vi "多路CAN初始化.vi"(8 "错误输入（无错误）":errorcluster, 11 "CAN通道in":u16[](array[numeric])=[81, 82, 83]) -> (0 "错误out（无错误）":errorcluster caption="错误输入（无错误）", 3 "CAN 通道out":u16[](array[numeric]))   [LabVIEW 2020]
uses:
  <userlib>/PCANBasic/PCANBasic.lvlib
panel:
  out "function return":u32 format="%.0x"
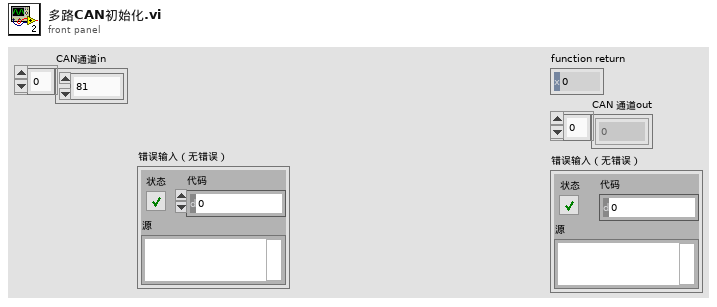
[diagram p1: front panel]
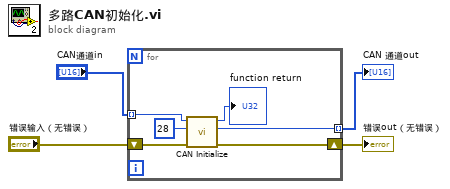
[diagram p0: block diagram]
diagram:
  n1 = for {
    tunnel: "CAN通道in" -> [w10] mode=indexing
    tunnel: [w7] -> w3 mode=indexing
    shift-right: [w5] -> w1
    shift-left: "错误输入（无错误）" -> [w6]
    n2 = call <userlib>:"CAN Initialize.vi"("错误输入（无错误）"=w6, "Btr0Btr1"=u16 28, "Channel"=w10) -> ("错误输出"=w5:errorcluster, "Channel out"=w7:u16, "function return"=→"function return":u32)  [unwired: 6 in]
  }
  "CAN 通道out" <- w3
  "错误out（无错误）" <- w1
